vi "init temp chart property nodes.vi"(1 "Temperature History":refnum<vi>, 7 "Power control visible":bool, 12 "range indicators":refnum<vi>[](array[refnum]), 14 "Power Control":refnum<vi>) -> ()   [LabVIEW 2014]
doc: "This subvi inits various properties for the temperature controller\n\nPaul K Dixon\nPhysics 350\nPaul K Dixon"
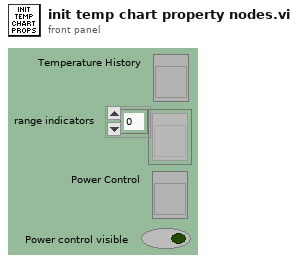
[diagram p1: front panel]
types:
  T1 = cluster{"Element Data":dbl, "Element Data":dbl, "Element Data":dbl, "Element Data":dbl, "Element Data":dbl, "Element Data":dbl, "Element Data":dbl}
  T2 = cluster{"Element Data":dbl, "Element Data":dbl, "Element Data":dbl, "Element Data":dbl, "Element Data":dbl, "Element Data":dbl, "Element Data":dbl}[]
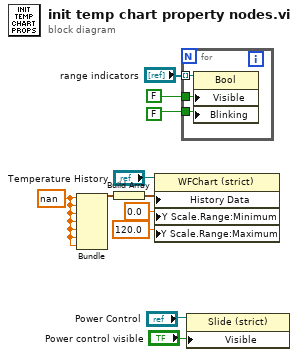
[diagram p0: block diagram]
diagram:
  w3 = nan ("Element Data")
  n1 = Bundle("Element Data"=w3, "Element Data"=w3, "Element Data"=w3, "Element Data"=w3, "Element Data"=w3, "Element Data"=w3, "Element Data"=w3) -> (w8:T1)  [unwired: 1 out]
  n2 = Build Array(w8) -> (w7:T2)
  n3 = property class="WFChart (strict)"(reference="Temperature History", "History Data"=w7, "Y Scale.Range:Minimum"=0.0, "Y Scale.Range:Maximum"=120.0) -> ()  [unwired: 1 in, 2 out]
  n4 = for {
    tunnel: "range indicators" -> [w14] mode=indexing
    tunnel: FALSE ("Visible") -> [w13]
    tunnel: FALSE ("Visible") -> [w12]
    n5 = property class="Bool"(reference=w14, "Visible"=w12, "Blinking"=w13) -> ()  [unwired: 1 in, 2 out]
  }
  n6 = property class="Slide (strict)"(reference="Power Control", "Visible"="Power control visible") -> ()  [unwired: 1 in, 2 out]
